vi "Edit Line.vi"(8 "error in":errorcluster, 10 "Line Name":string, 11 "References":T1) -> (0 "error out":errorcluster, 2 "change?":bool)   [LabVIEW 2014, in "DAQmx Module editor node.lvclass"]
doc: "This VI edits the properties of a line. It will unlink channels and tags and create new links to channels and tags."
uses:
  DAQmx Module editor node.lvclass
  <vilib>/NI/DCAF/Tag Editor Core/Table API/Table Manager/object ref.ctl
  <vilib>/NI/DCAF/Tag Editor Core/Configuration Editor/Classes/Engine Parent/Engine Parent Editor Node.lvclass
  <vilib>/NI/DCAF/Tag Editor Core/Configuration Editor/Classes/Module editor node/module editor node.lvclass
  module/configuration/DAQmx Module Configuration.lvclass
  module/configuration/DAQmx Module Configuration.lvclass/DAQmx Module Configuration.ctl
  <vilib>/NI/Configuration Framework/serializable configuration/NISE_CEF_serializable configuration.lvclass/NISE_CEF_serializable configuration.ctl
  <vilib>/Utility/LVClass/Get LV Class Name.vi
  <vilib>/NI/Configuration Framework/error generator/NISE_error generator.vi
  <vilib>/NI/Tag Bus Module Framework/channel/TBM channel.lvclass
  <vilib>/NI/Configuration Framework/serializable configuration/NISE_CEF_serializable configuration.lvclass
  <vilib>/NI/DCAF/Tag Editor Core/Table API/Table Manager/Table Manager.lvclass
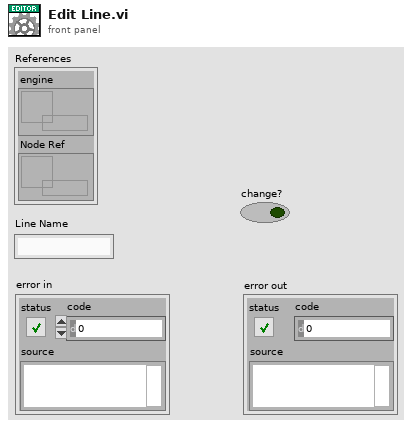
[diagram p1: front panel]
types:
  T1 = typedef "Table Manager.lvlib/Table Manager.lvclass/object ref.ctl" = cluster{"engine":refnum<data-value>, "Node Ref":refnum<data-value>}
  T2 = typedef "DAQmx Module Configuration.lvclass/Line.ctl" = cluster{"channel":refnum<class "TBM channel.lvclass">, "Physical Channel":string, "Measurement Type":T3, "Parameters":T4}
  T3 = typedef "DAQmx Module Configuration.lvclass/Measurement Type.ctl" = enum16{"Digital Input", "Digital Output", "Voltage Input", "Voltage Output", "Current Input", "Current Output", "RTD", "Thermocouple", "Strain"}
  T4 = typedef "DAQmx Module Configuration.lvclass/Parameters.ctl" = cluster{"Digital Config":cluster{"Invert Lines?":bool}, "Voltage Config":cluster{"Maximum Value (V)":dbl, "Minimum Value (V)":dbl, "in terminal configuration (V)":i32, "out terminal configuration (V)":i32}, "Current Config":cluster{"Maximum Value (A)":dbl, "Minimum Value (A)":dbl, "shunt resistor location":i32, "input terminal configuration (C)":i32, "external shunt resistor value":dbl}, "RTD Config":cluster{"Maximum Value (°C)":dbl, "Minimum Value (°C)":dbl, "resistance configuration":i32, "r0":dbl, "current excitation value":dbl, "rtd type":i32, "current excitation source":i32}, "Thermocouple Config":cluster{"Minimum Value (C)":dbl, "Maximum Value (C)":dbl, "thermocouple type":i32, "cjc source":i32, "cjc value":dbl}, "Strain Config":cluster{"Maximum Value":dbl, "Minimum Value":dbl, "bridge information":cluster{"strain configuration":i32, "lead wire resistance":dbl, "initial bridge voltage":dbl, "voltage excitation source":i32, "voltage excitation value":dbl}, "strain gage information":cluster{"gage factor":dbl, "nominal gage resistance":dbl, "poisson ratio":dbl}}}
  T5 = typedef "DAQmx Module editor node.lvclass/Mappings.ctl" = cluster{"Line":T2, "Maps":T6[]}
  T6 = typedef "DAQmx Module editor node.lvclass/Map.ctl" = cluster{"channel":refnum<class "TBM channel.lvclass">, "tag name":string}
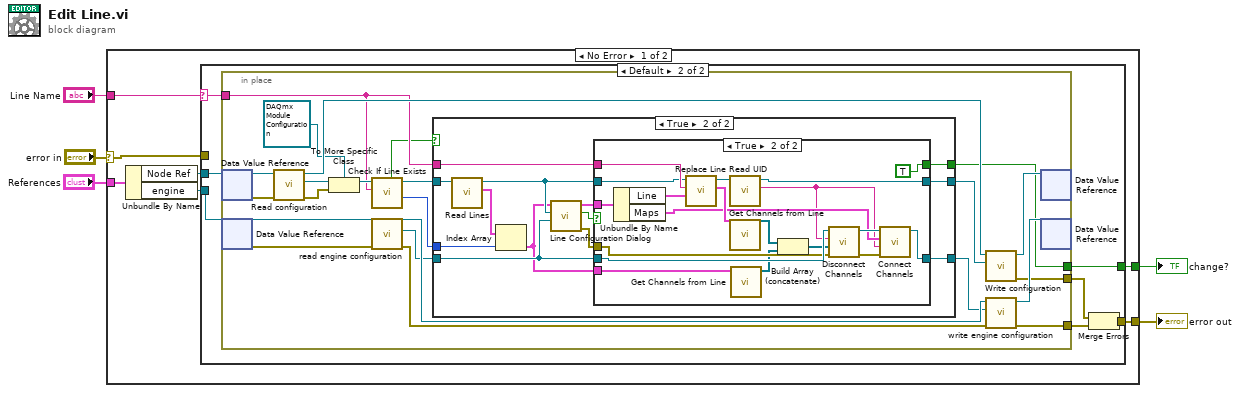
[diagram p0: block diagram]
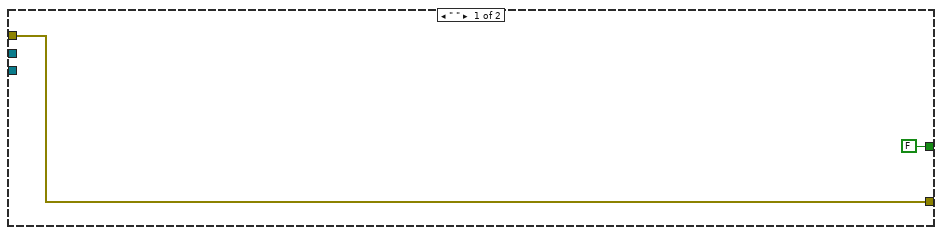
[diagram p2: hidden frame]
diagram:
  n1 = case shown="No Error" "error in" {
    selector: "error in" -> [w6 w81]
    tunnel: "References" -> [w10 _]
    tunnel: "Line Name" -> [w7 _]
    tunnel: [w9 w81] -> w2
    tunnel: [w8 _] -> w1
    frame No Error {
      n2 = Unbundle By Name(w10) -> ("Node Ref"=w12:refnum<data-value>, "engine"=w11:refnum<data-value>)
      n3 = case shown="Default" w7 {
        selector: w7 -> [_ w15]
        tunnel: w12 -> [_ w21]
        tunnel: w11 -> [_ w20]
        tunnel: [w13 w17] -> w9
        tunnel: [FALSE ("change?") w16] -> w8
        tunnel: w6 -> [w13 _]
        frame " " {
        }
        frame Default {
          n4 = in-place {
            in-place-border: [w25] -> w19
            in-place-border: [w41] -> w18
            in-place-border: [w24] -> w16
            in-place-border: w15 -> [w30]
            n5 = in-place-dvr #1(w21) -> (w37:refnum<class "module editor node.lvclass">, w31:errorcluster)
            n6 = in-place-dvr #2(w20) -> (w44:refnum<class "Engine Parent Editor Node.lvclass">, w43:errorcluster)
            n7 = call-dynamic "Read configuration.vi"("error in"=w31, "NISE_CEF_serializable node in"=w37) -> ("error out"=w34:errorcluster, "configuration"=w35:refnum<class "NISE_CEF_serializable configuration.lvclass">, "NISE_CEF_serializable node out"=w36:refnum<class "module editor node.lvclass">)  [unwired: 7 in]
            n8 = To More Specific Class(target class=refnum<class "DAQmx Module Configuration.lvclass"> refnum ("tag bus configurable plugin module configuration"), reference=w35, error in=w34) -> (specific class reference=w32:refnum<class "DAQmx Module Configuration.lvclass">)  [unwired: 1 out]
            n9 = call-dynamic "Check If Line Exists.vi"("Name to Locate"=w30, "Daqmx Module configuration in"=w32) -> ("Index"=w27:i32, "Daqmx Module configuration out"=w28:refnum<class "DAQmx Module Configuration.lvclass">, "Found?"=w22:bool)  [unwired: 5 in, 2 out]
            n10 = call <vilib>:"read engine configuration.vi"("error in"=w43, "Engine Parent Editor Node in"=w44) -> ("error out"=w39:errorcluster, "engine configuration"=w26:refnum<class "engine configuration.lvclass">, "Engine Parent Editor Node out"=w40:refnum<class "Engine Parent Editor Node.lvclass">)  [unwired: 7 in]
            n11 = case shown="True" w22 {
              tunnel: w28 -> [w46 w57]
              tunnel: w26 -> [w45 w48]
              tunnel: w30 -> [_ w59]
              tunnel: [w46 w52] -> w29
              tunnel: w27 -> [_ w54]
              tunnel: [_ w50] -> w24
              tunnel: [w45 w49] -> w23
              frame False {
              }
              frame True {
                n12 = call "Read Lines.vi"("Daqmx Module configuration in"=w57) -> ("Lines"=w55:T2[], "Daqmx Module configuration out"=w56:refnum<class "DAQmx Module Configuration.lvclass">)  [unwired: 8 in, 1 out]
                n13 = Index Array(array=w55, index=w54) -> (element=w47:T2)
                n14 = call "Line Configuration Dialog.vi"("engine configuration in"=w48, "tag bus configurable plugin module configuration"=w56, "Line"=w47) -> ("error out"=w58:errorcluster, "changed"=w51:bool, "Mappings out"=w53:T5)  [unwired: 5 in, 1 out]
                n15 = case shown="True" w51 {
                  tunnel: w59 -> [_ w80]
                  tunnel: w48 -> [w60 w79]
                  tunnel: w58 -> [_ w78]
                  tunnel: w56 -> [w61 w74]
                  tunnel: w53 -> [_ w73]
                  tunnel: [w61 w71] -> w52
                  tunnel: [_ TRUE ("change?")] -> w50
                  tunnel: [w60 w65] -> w49
                  tunnel: w47 -> [_ w62]
                  frame False {
                  }
                  frame True {
                    n16 = Unbundle By Name(w73) -> ("Line"=w72:T2, "Maps"=w68:T6[])
                    n17 = call "Replace Line.vi"("New Line"=w72, "Line Name"=w80, "Daqmx Module configuration in"=w74) -> ("Old Line"=w76:T2, "Daqmx Module configuration out"=w77:refnum<class "DAQmx Module Configuration.lvclass">)  [unwired: 6 in, 1 out]
                    n18 = call <vilib>:"Read UID.vi"("configuration in"=w77) -> ("instance id"=w67:string, "configuration out"=w71:refnum<class "DAQmx Module Configuration.lvclass">)  [unwired: 8 in, 1 out]
                    n19 = call "Get Channels from Line.vi"("Line"=w76) -> ("Channels"=w75:refnum<class "TBM channel.lvclass">[])  [unwired: 10 in]
                    n20 = call "Get Channels from Line.vi"("Line"=w62) -> ("Channels"=w63:refnum<class "TBM channel.lvclass">[])  [unwired: 10 in]
                    n21 = Build Array (concatenate)(w75, w63) -> (w64:refnum<class "TBM channel.lvclass">[])
                    n22 = call "Disconnect Channels.vi"("error in (no error)"=w78, "Deleted Channels"=w64, "instance id"=w67, "Engine Configuration in"=w79) -> ("error out"=w69:errorcluster, "Engine Configuration out"=w70:refnum<class "engine configuration.lvclass">)  [unwired: 6 in]
                    n23 = call "Connect Channels.vi"("error in (no error)"=w69, "instance id"=w67, "Maps"=w68, "Engine Configuration in"=w70) -> ("Engine Configuration out"=w65:refnum<class "engine configuration.lvclass">)  [unwired: 6 in, 1 out]
                  }
                }
              }
            }
            n24 = call-dynamic "Write configuration.vi"("configuration"=w29, "NISE_CEF_serializable node in"=w36) -> ("error out"=w25:errorcluster, "NISE_CEF_serializable node out"=w38:refnum<class "module editor node.lvclass">)  [unwired: 8 in]
            n25 = call <vilib>:"write engine configuration.vi"("error in"=w39, "engine configuration"=w23, "Engine Parent Editor Node in"=w40) -> ("error out"=w41:errorcluster, "Engine Parent Editor Node out"=w42:refnum<class "Engine Parent Editor Node.lvclass">)  [unwired: 7 in]
            n26 = in-place-dvr #1(w38) -> ()  [unwired: 2 out]
            n27 = in-place-dvr #2(w42) -> ()  [unwired: 2 out]
          }
          n28 = Merge Errors(w19, w18) -> (w17:errorcluster)
        }
      }
    }
    frame Error {
    }
  }
  "change?" <- w1
  "error out" <- w2
